vi "Actor Core.vi"(8 "error in":errorcluster, 11 "HIJ Multiple Cams App Demo In":refnum<class "HIJ 4 Alignment Cams App.lvclass">) -> (0 "error out":errorcluster, 3 "Actor out":refnum<class "Actor.lvclass">)   [LabVIEW 2014, in "HIJ 4 Alignment Cams App.lvlib" / "HIJ 4 Alignment Cams App.lvclass"]
doc: "(<B>Filename</B>: Actor Framework.lvlib:Actor.lvclass:Actor Core.vi)\n\nReceives messages to the actor, reacts to them, and initiates any error handling that may shut the actor down.\n\nDescendant classes may override this VI to append parallel tasks for the actor to complete while it handles messages. Overrides use the Call Parent Method node."
uses:
  HIJ 4 Alignment Cams App.lvclass
  <vilib>/ActorFramework/Actor/Actor.lvclass
  HIJ Vision App IMAQdx Display/HIJ Vision App IMAQdx Display/HIJ Vision App IMAQdx Display.lvclass
  Analyze/Results and Overlays/Static Text Overlay/Static Text Overlay.lvclass
  Analyze/Results and Overlays/Static Overlay/Static Position.ctl
  Display Actors/HIJ IMAQdx Display/AF IMAQ Display/HIJ IMAQdx Display.lvclass
  Analyze/Results and Overlays/Static Overlay/Static Overlay.lvclass/Static Overlay.ctl
  HIJ 4 Alignment Cams App.lvclass/HIJ 4 Alignment Cams App.ctl
  Display Actors/HIJ Vision Display/HIJ Vision Display/HIJ Vision Display.lvclass/HIJ Vision Display.ctl
  Display Actors/HIJ IMAQdx Display/AF IMAQ Display/HIJ IMAQdx Display.lvclass/HIJ IMAQdx Display.ctl
  HIJ Vision App IMAQdx Display/HIJ Vision App IMAQdx Display/HIJ Vision App IMAQdx Display.lvclass/HIJ Vision App IMAQdx Display.ctl
  CamAppInfo.ctl
  <vilib>/userdefined/High Color/IMAQdx.ctl
  <vilib>/ActorFramework/Message Enqueuer/Message Enqueuer.lvclass
  Analyze/Results and Overlays/Static Text Overlay/Static Text Overlay.lvclass/Static Text Overlay.ctl
  Shared Code/Viewable Actor/ViewableActor Messages/Insert Into SubPanel Msg/Insert Into SubPanel Msg.lvclass/Insert Into SubPanel Msg.ctl
  <vilib>/ActorFramework/Message Enqueuer/Message Enqueuer.lvclass/Message Enqueuer.ctl
  <vilib>/ActorFramework/Actor/Actor.lvclass/Actor.ctl
  HIJ 4 Alignment Cams App Messages/Exchange Main Camera Msg/Exchange Main Camera Msg.lvclass/Exchange Main Camera Msg.ctl
  HIJ 4 Alignment Cams App Messages/Forward Menu Selection Msg/Forward Menu Selection Msg.lvclass/Forward Menu Selection Msg.ctl
  HIJ 4 Alignment Cams App Messages/Menu Activation Msg/Menu Activation Msg.lvclass/Menu Activation Msg.ctl
  Analyze/Results and Overlays/Static Text Overlay/Write OVL Text.vi
  Analyze/Results and Overlays/Static Overlay/Write Static Position.vi
  Display Actors/HIJ Vision Display/HIJ Vision Display/Write WorkDir.vi
  Display Actors/HIJ IMAQdx Display/AF IMAQ Display/Write ConfigDir.vi
  HIJ Vision App IMAQdx Display/HIJ Vision App IMAQdx Display/Write Caller Menu Ref.vi
  <vilib>/ActorFramework/Message Enqueuer/Enqueue.vi
  <vilib>/ActorFramework/Message Enqueuer/Init from Existing Queue.vi
  Application Base Actors/HIJ Vision Camera App/HIJ Vision Camera App/Write my WorkDir.vi
  Application Base Actors/HIJ Vision Camera App/HIJ Vision Camera App/Write my ConfigDir.vi
  Application Base Actors/HIJ Vision Camera App/HIJ Vision Camera App/Write Start Acquisition.vi
  Application Base Actors/HIJ Vision Application/HIJ Vision Application/Write HIJ Vision Display.vi
  Application Base Actors/HIJ Vision Camera App/HIJ Vision Camera App/Write Start Camera.vi
  <vilib>/ActorFramework/Message Priority Queue/Priority Enqueue.vi
  Shared Code/Viewable Actor/ViewableActor Messages/Insert Into SubPanel Msg/Insert Into SubPanel Msg.lvclass
  HIJ 4 Alignment Cams App Messages/Exchange Main Camera Msg/Exchange Main Camera Msg.lvclass
  HIJ 4 Alignment Cams App Messages/Forward Menu Selection Msg/Forward Menu Selection Msg.lvclass
  HIJ 4 Alignment Cams App Messages/Menu Activation Msg/Menu Activation Msg.lvclass
  <vilib>/ActorFramework/Stop Msg/Stop Msg.lvclass
  Shared Code/Viewable Actor/ViewableActor/ViewableActor.lvclass
  Analyze/Results and Overlays/Static Overlay/Static Overlay.lvclass
panel:
  in  "Stop Button":bool
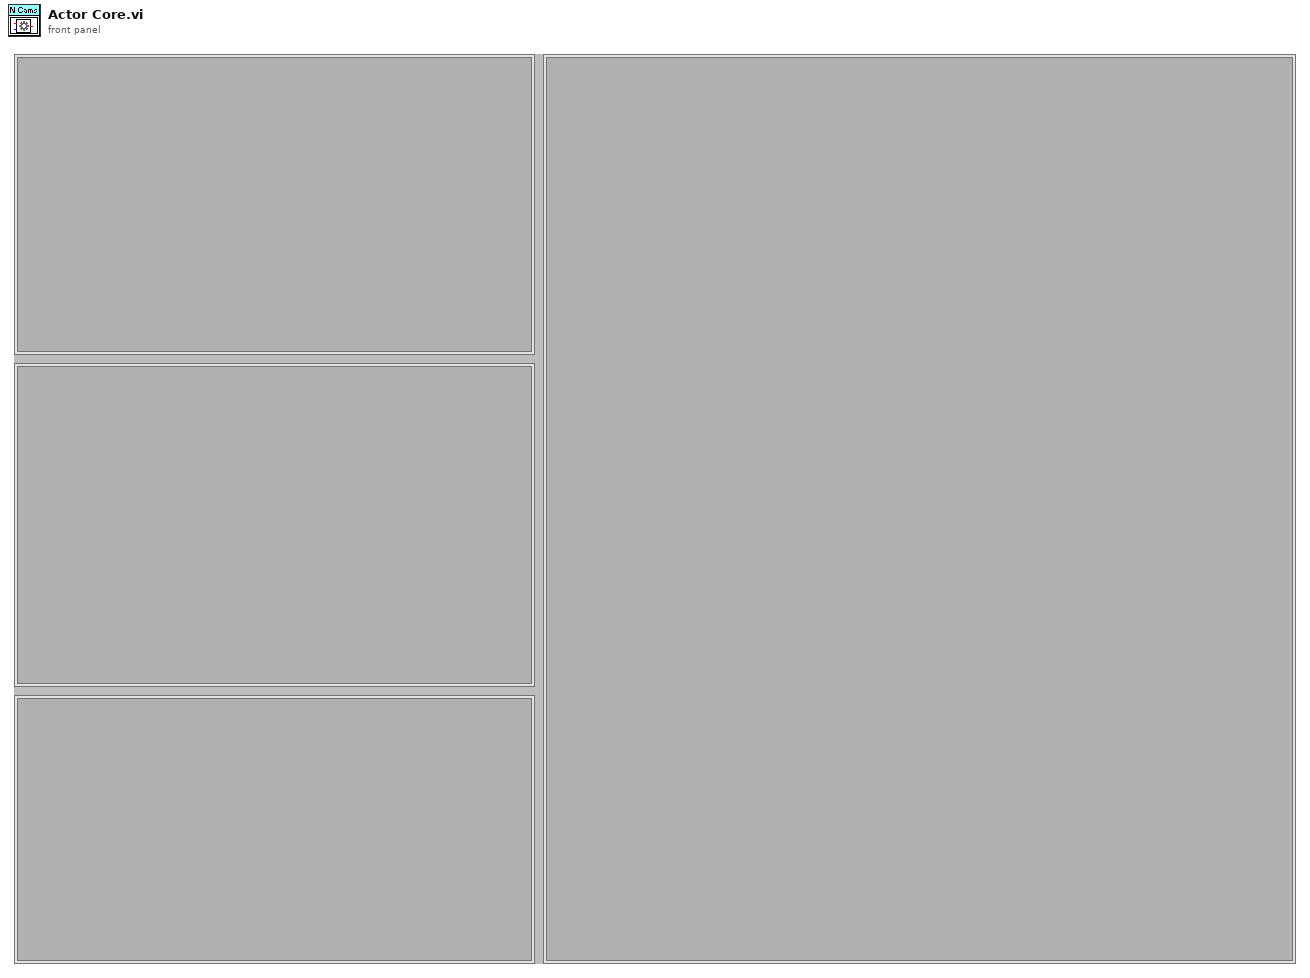
[diagram p1: front panel]
types:
  T1 = typedef "Static Overlay.lvclass/Static Position.ctl" = enum16{"Top Left", "Top Center", "Top Right", "Center", "Bottom Left", "Bottom Center", "Bottom Right"}
  T2 = cluster{"Desired Font (Application)":enum16{"User-specified Font", "Application Font", "System Font", "Dialog Font"}, "[User-specified Font]":cluster{"Font Name":string, "Size":i16, "Strikeout?":bool, "Italic?":bool, "Underline?":bool, "Outline?":bool, "Shadow?":bool, "Bold?":bool, "Rotation Angle":dbl}, "Horizontal Alignment":i16, "Vertical Alignment":i16}
  T3 = typedef "IMAQdx.ctl" = refnum<k21>
  T4 = typedef "HIJ 4 Alignment Cams App.lvlib/HIJ 4 Alignment Cams App.lvclass/CamAppInfo.ctl" = cluster{"Camera":T3, "App enq":refnum<class "Message Enqueuer.lvclass">, "SubPnl Refnum":refnum<vi>}
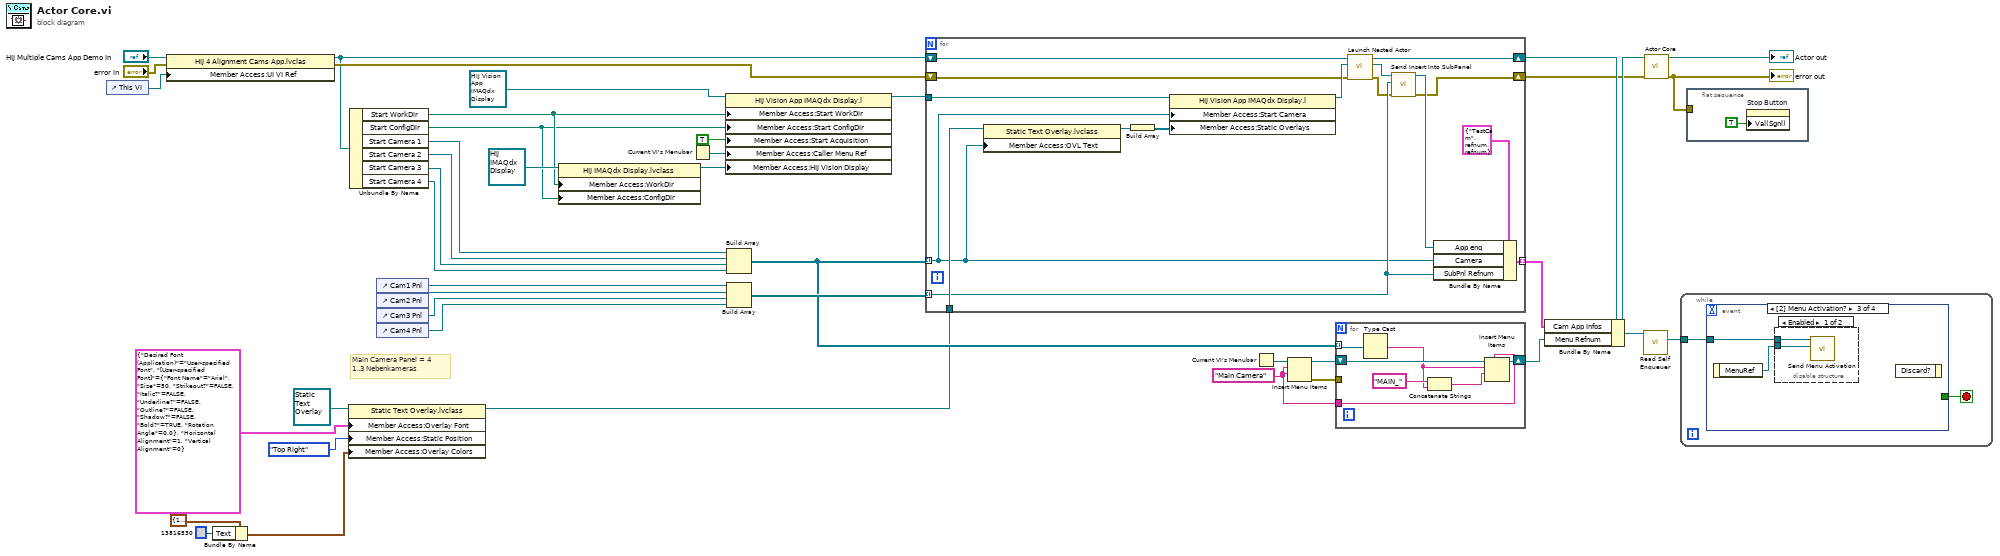
[diagram p0: block diagram]
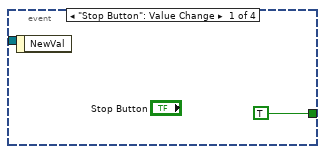
[diagram p2: hidden frame]
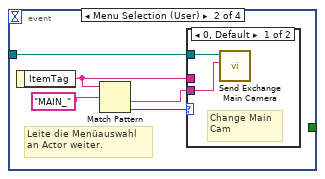
[diagram p3: hidden frame]
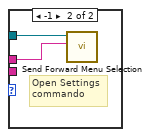
[diagram p4: hidden frame]
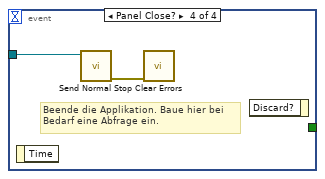
[diagram p6: hidden frame]
diagram:
  w13 = "Main Camera" ("menu tag")
  # "Main Camera Panel = 4\n1..3 Nebenkameras"
  n1 = control-ref of="This VI"() -> (w37:refnum<vi>)
  n2 = property class="HIJ 4 Alignment Cams App.lvclas"(reference="HIJ Multiple Cams App Demo In", error in="error in", "Member Access:UI VI Ref"=w37) -> (reference out=w33:refnum<class "HIJ 4 Alignment Cams App.lvclass">, error out=w35:errorcluster)
  n3 = Bundle By Name(cluster=cluster{"Border":u32, "Text":u32} {"Border"=16448250, "Text"=16448250} ("Overlay Colors"), "Text"=u32 13816530) -> (w6:cluster{"Border":u32, "Text":u32})
  n4 = property class="Static Text Overlay.lvclass"(reference=refnum<class "Static Text Overlay.lvclass"> refnum ("Static Text Overlay.lvclass"), "Member Access:Overlay Font"=T2 {"Desired Font (Application)"=enum."User-specified Font", "[User-specified Font]"={"Font Name"="Arial", "Size"=50, "Strikeout?"=FALSE, "Italic?"=FALSE, "Underline?"=FALSE, "Outline?"=FALSE, "Shadow?"=FALSE, "Bold?"=TRUE, "Rotation Angle"=0.0}, "Horizontal Alignment"=1, "Vertical Alignment"=0} ("Overlay Font"), "Member Access:Static Position"=Static_Position."Top Right" ("Static Position"), "Member Access:Overlay Colors"=w6) -> (reference out=w10:refnum<class "Static Text Overlay.lvclass">)  [unwired: 1 in, 1 out]
  n5 = Unbundle By Name(w33) -> ("Start WorkDir"=w3:path, "Start ConfigDir"=w2:path, "Start Camera 1"=w30:T3, "Start Camera 2"=w29:T3, "Start Camera 3"=w28:T3, "Start Camera 4"=w27:T3)
  n6 = control-ref of="Cam1 Pnl"() -> (w24:refnum<vi>)
  n7 = control-ref of="Cam2 Pnl"() -> (w23:refnum<vi>)
  n8 = control-ref of="Cam3 Pnl"() -> (w22:refnum<vi>)
  n9 = control-ref of="Cam4 Pnl"() -> (w21:refnum<vi>)
  n10 = property class="HIJ IMAQdx Display.lvclass"(reference=refnum<class "HIJ IMAQdx Display.lvclass"> refnum ("HIJ IMAQdx Display.lvlib:HIJ IMAQdx Display.lvclass"), "Member Access:WorkDir"=w3, "Member Access:ConfigDir"=w2) -> (reference out=w1:refnum<class "HIJ IMAQdx Display.lvclass">)  [unwired: 1 in, 1 out]
  n11 = Current VI's Menubar() -> (w32:refnum<k9>)
  n12 = property class="HIJ Vision App IMAQdx Display.l"(reference=refnum<class "HIJ Vision App IMAQdx Display.lvclass"> refnum ("HIJ Vision App IMAQdx Display.lvlib:HIJ Vision App IMAQdx Display.lvclass"), "Member Access:Start WorkDir"=w3, "Member Access:Start ConfigDir"=w2, "Member Access:Start Acquisition"=TRUE ("Start Acquisition"), "Member Access:Caller Menu Ref"=w32, "Member Access:HIJ Vision Display"=w1) -> (reference out=w31:refnum<class "HIJ Vision App IMAQdx Display.lvclass">)  [unwired: 1 in, 1 out]
  n13 = Build Array(w30, w29, w28, w27) -> (w14:T3[])
  n14 = Build Array(w24, w23, w22, w21) -> (w20:refnum<vi>[])
  n15 = for {
    tunnel: w31 -> [w44]
    shift-right: [w49] -> w25
    shift-left: w35 -> [w54]
    shift-right: [w52] -> w34
    shift-left: w33 -> [w50]
    tunnel: w20 -> [w55] mode=indexing
    tunnel: w14 -> [w46] mode=indexing
    tunnel: [w48] -> w19 mode=indexing
    tunnel: w10 -> [w58]
    n16 = property class="Static Text Overlay.lvclass"(reference=w58, "Member Access:OVL Text"=w46) -> (reference out=w45:refnum<class "Static Text Overlay.lvclass">)  [unwired: 1 in, 1 out]
    n17 = Build Array(w45) -> (w43:refnum<class "Static Text Overlay.lvclass">[])
    n18 = property class="HIJ Vision App IMAQdx Display.l"(reference=w44, "Member Access:Start Camera"=w46, "Member Access:Static Overlays"=w43) -> (reference out=w57:refnum<class "HIJ Vision App IMAQdx Display.lvclass">)  [unwired: 1 in, 1 out]
    n19 = call <vilib>:"Launch Nested Actor.vi"("error in (no error)"=w54, "Nested Actor"=w57, "Caller Actor in"=w50) -> ("error out"=w51:errorcluster, "Nested Actor's Enqueuer"=w53:refnum<class "Message Enqueuer.lvclass">, "Caller Actor out"=w52:refnum<class "HIJ 4 Alignment Cams App.lvclass">)  [unwired: 6 in]
    n20 = call "Send Insert Into SubPanel.vi"("error in (no error)"=w51, "SubPanel Ref"=w55, "Message Enqueuer"=w53) -> ("error out"=w49:errorcluster, "Message Enqueuer out"=w56:refnum<class "Message Enqueuer.lvclass">)  [unwired: 7 in]
    n21 = Bundle By Name(cluster=T4 {"Camera"="TestCam", "App enq"=refnum, "SubPnl Refnum"=refnum} ("Cam app info"), "App enq"=w56, "Camera"=w46, "SubPnl Refnum"=w55) -> (w48:T4)
  }
  n22 = Current VI's Menubar() -> (w17:refnum<k9>)
  n23 = Insert Menu Items(7:w13, 8:w13, 9:w17) -> (0:w15:errorcluster, 3:w16:refnum<k9>)  [unwired: 3 in, 1 out]
  n24 = for {
    tunnel: w15 -> [_]
    tunnel: w14 -> [w65] mode=indexing
    tunnel: w13 -> [w64]
    shift-right: [w59] -> w12
    shift-left: w16 -> [w61]
    n25 = Type Cast(x=w65) -> (*(type *) &x=w60:string)  [unwired: 1 in]
    n26 = Concatenate Strings("MAIN_" ("menu tag"), w60) -> (w62:string)
    n27 = Insert Menu Items(5:w64, 7:w62, 8:w60, 9:w61) -> (3:w59:refnum<k9>)  [unwired: 2 in, 2 out]
  }
  n28 = Bundle By Name(cluster=w34, "Cam App Infos"=w19, "Menu Refnum"=w12) -> (w26:refnum<class "HIJ 4 Alignment Cams App.lvclass">)
  n29 = call <vilib>:"Read Self Enqueuer.vi"("Actor"=w26) -> ("Self Enqueuer"=w40:refnum<class "Message Enqueuer.lvclass">)  [unwired: 10 in]
  n30 = call-parent "Actor Core.vi"("error in"=w25, "Actor in"=w26) -> ("error out"=w41:errorcluster, "Actor out"=→"Actor out":refnum<class "Actor.lvclass">)  [unwired: 8 in]
  "error out" <- w41
  n31 = while {
    tunnel: w40 -> [w66]
    stop <- w67 stop-if-true
    n32 = event shown="[2] Menu Activation?" {
      selector: _ -> [_ _ _ _]
      dyn-events: _ -> [_ _ _ _]
      timeout: _ -> [_ _ _ _]
      tunnel: [TRUE _ _ _] -> w67
      tunnel: w66 -> [_ w73 w79 w83]
      event "Stop Button": Value Change {
        n33 = event-data() -> ()  [unwired: 1 in, 1 out]
      }
      event Menu Selection (User) {
        # "Leite die Menüauswahl \nan Actor weiter."
        n34 = event-data() -> ("ItemTag"=w72:string)  [unwired: 1 in]
        n35 = Match Pattern(string=w72, regular expression="MAIN_" ("menu tag")) -> (after substring=w69:string, offset past match=w70:i32)  [unwired: 1 in, 2 out]
        n36 = case shown="0, Default" w70 {
          tunnel: w73 -> [w75 w77]
          tunnel: w72 -> [_ w76]
          tunnel: w69 -> [w74 _]
          frame 0, Default {
            # "Change Main\nCam"
            n37 = call "Send Exchange Main Camera.vi"("New Main Cam"=w74, "Message Enqueuer"=w75) -> ()  [unwired: 8 in, 2 out]
          }
          frame -1 {
            # "Open Settings\ncommando"
            n38 = call "Send Forward Menu Selection.vi"("MenuTag"=w76, "Message Enqueuer"=w77) -> ()  [unwired: 8 in, 2 out]
          }
        }
      }
      event Menu Activation? {
        n39 = event-data() -> ("MenuRef"=w78:refnum<k9>)  [unwired: 1 in]
        n40 = disable-structure shown="Enabled" {
          disable-tunnel: w79 -> [w81 _]
          disable-tunnel: w78 -> [w80 _]
          frame Enabled {
            n41 = call "Send Menu Activation.vi"("Menu Refnum"=w80, "Message Enqueuer"=w81) -> ()  [unwired: 8 in, 2 out]
          }
          frame Disabled {
          }
        }
        n42 = event-data() -> ()  [unwired: 2 in, 1 out]
      }
      event Panel Close? {
        # "Beende die Applikation. Baue hier bei\nBedarf eine Abfrage ein."
        n43 = event-data() -> ()  [unwired: 1 in, 1 out]
        n44 = call <vilib>:"Send Normal Stop.vi"("Message Enqueuer"=w83) -> ("error out"=w82:errorcluster)  [unwired: 10 in]
        n45 = call <vilib>:"Clear Errors.vi"("error in (no error)"=w82) -> ()  [unwired: 5 in, 2 out]
        n46 = event-data() -> ()  [unwired: 2 in, 1 out]
      }
    }
  }
  n47 = flat-sequence {
    tunnel: w41 -> [_]
    frame #0 {
      n48 = property on="Stop Button" class="Bool (strict)"("Val(Sgnl)"=TRUE) -> ()  [unwired: 2 in, 2 out]
    }
  }
